vi "Deterministic Errors.New Allocated String.vi"   [LabVIEW 2016, in "Deterministic Errors.lvlib"]
uses:
  Deterministic Errors.lvlib
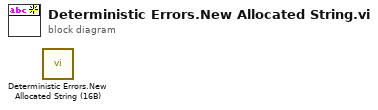
[diagram p0: block diagram]
diagram:
  n1 = call "Deterministic Errors.New Allocated String (16B).vi"() -> ()  [unwired: 11 in, 1 out]
